vi "TazeASharg - Copy.vi"() -> ()   [LabVIEW 2022 SP3]
uses:
  StopControl.ctl
  StartControl.ctl
  ScoreIndicator.ctl
  TimeControl.ctl
  ComboIndicator.ctl
  NameControl.ctl
  FullHighscoreIndicator.ctl
  HighscoreIndicator.ctl
  FullHighScoreScoreIndicator.ctl
  HighscoreIndicatorYes.ctl
  ShargStates.ctl
  ShargTypeDef.ctl
  <vilib>/numeric/Random Number (Range) U64.vi
  <vilib>/numeric/sub_Random U32.vi
  <vilib>/MakerHub/LINX/Public/Utilities/Open Serial.vi
  <vilib>/MakerHub/LINX/Public/Sensors/Motion/Servo/Servo Open One Channel.vi
  <vilib>/MakerHub/LINX/Public/Sensors/Motion/Servo/Servo Close One Channel.vi
  <vilib>/MakerHub/LINX/LMH-LINX.lvlib
  <vilib>/MakerHub/LINX/Public/Sensors/Motion/Servo/Servo.lvlib
  <vilib>/MakerHub/LINX/Public/Peripherals/PWM/PWM Set Duty Cycle N Chans.vi
panel:
  out "High Score Scores":T1 caption="HIGH SCORE"
  out "High Score Names":T3 caption="HIGH SCORE"
  in  "Name":T5 caption="NAME"
  out "Overheat":bool
  out "COMBO":T6 format="%01d"
  out "TIME":T7 format="%02d"
  out "Hit?":bool
  out "SCORE":T8 format="%04d"
  in  "Start Game":T9
  in  "Stop Button":T10
  out "Energy":dbl(knob) caption="LASER ENERGY" scale=0.0..180.0
  # "HIGH SCORE"
  # "1."
  # "2."
  # "3."
  # "4."
  # "5."
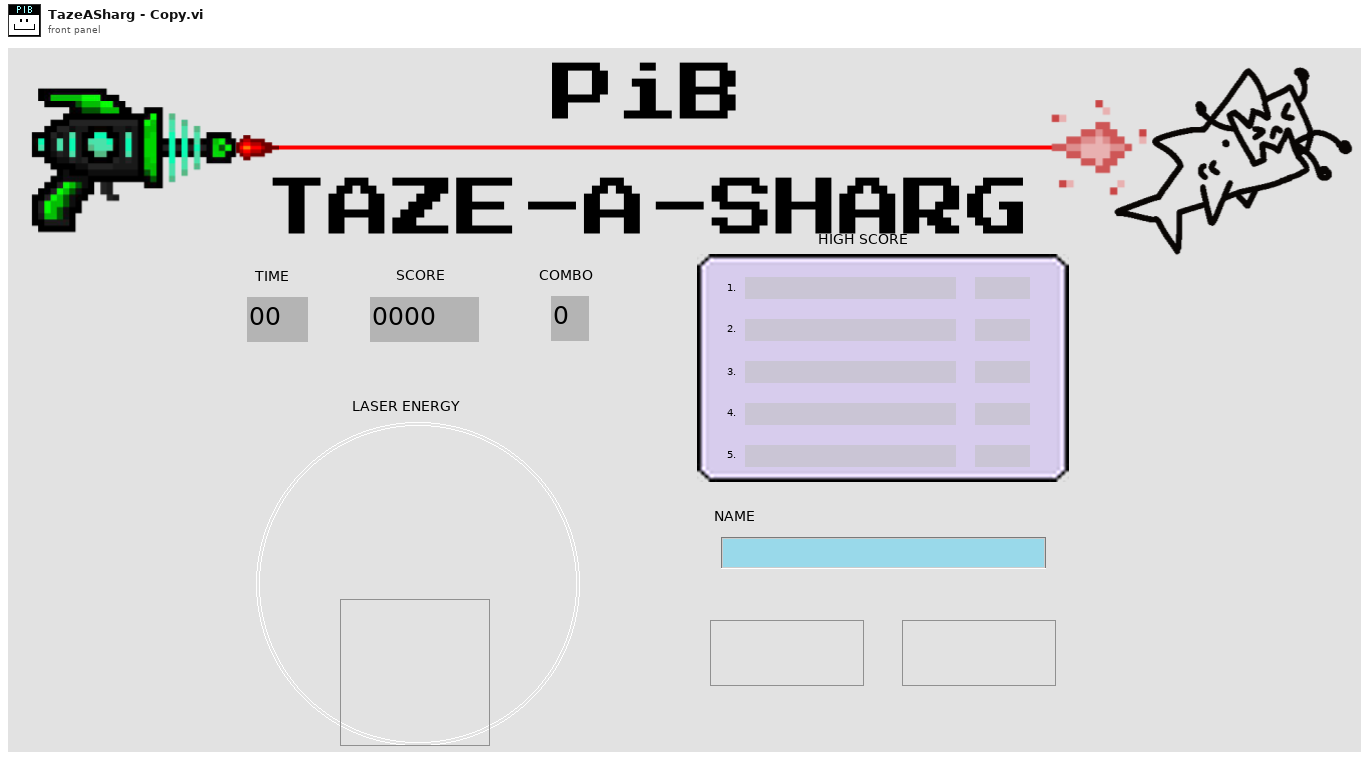
[diagram p1: front panel]
types:
  T1 = typedef "FullHighScoreScoreIndicator.ctl" = T2[]
  T2 = typedef "HighscoreIndicatorYes.ctl" = string
  T3 = typedef "FullHighscoreIndicator.ctl" = T4[]
  T4 = typedef "HighscoreIndicator.ctl" = string
  T5 = typedef "NameControl.ctl" = string
  T6 = typedef "ComboIndicator.ctl" = u32
  T7 = typedef "TimeControl.ctl" = u32
  T8 = typedef "ScoreIndicator.ctl" = u32
  T9 = typedef "StartControl.ctl" = bool
  T10 = typedef "StopControl.ctl" = bool
  T11 = cluster{"Target Up":bool, "Target Start Time":u32, "Target Up Time":u64, "Current Target":u64}
  T12 = cluster{"Laser Pin":u8, "Trigger Pin":u8, "Servo Pin":u8, "Photoresistor Pins":u8[], "RGB LED Pins":u8[]}
  T13 = typedef "ShargStates.ctl" = enum16{"Initialization", "Leaderboard", "Start Game", "Gameplay", "Update Final Score"}
  T14 = typedef "LMH-LINX.lvlib/LINX Ref.ctl" = cluster{"IO":T15, "Interface":T16, "LINX Device Config":T17}
  T15 = typedef "LMH-LINX.lvlib/Platform.ctl" = enum16{"Remote", "Local"}
  T16 = typedef "LMH-LINX.lvlib/Interface.ctl" = enum16{"Serial", "TCP"}
  T17 = typedef "LMH-LINX.lvlib/Device.lvlib/LINX Device Config.ctl" = cluster{"Interface":T16, "COM Port":refnum<visa-resource-name>, "TCP Configuration":T18, "Device Family":u8, "Device ID":u8, "Device Name":string, "TCP Ref":refnum<k5>, "Channels":T19}
  T18 = typedef "LMH-LINX.lvlib/Device.lvlib/TCP Config.ctl" = cluster{"IP Address":string, "Port":u16}
  T19 = typedef "LMH-LINX.lvlib/Channels.ctl" = cluster{"DI":u8[], "DO":u8[], "AI":u8[], "AO":u8[], "PWM":u8[], "QE":u8[], "UART":u8[], "I2C 2":u8[], "SPI":u8[], "CAN":u8[], "Servo":u8[], "AI Ref (V)":dbl, "AI Resolution (Bits)":u8, "AO Ref (V)":dbl, "AO Resolution (Bits)":u8}
  T20 = cluster{"Target Up":bool, "millisecond timer value":u32, "number":u64, "Current Target":u64}
  T21 = enum16{"open", "open or create", "create or replace", "create", "open (read-only)"}
  T22 = typedef "ShargTypeDef.ctl" = cluster{"Start Time":u32, "Score":u32, "Combo":u32, "RisingEdge":u32, "FallingEdge":u32, "Duration":u32, "Signal":i16, "NewTarget?":bool, "Username":string, "LastChannel":i32}
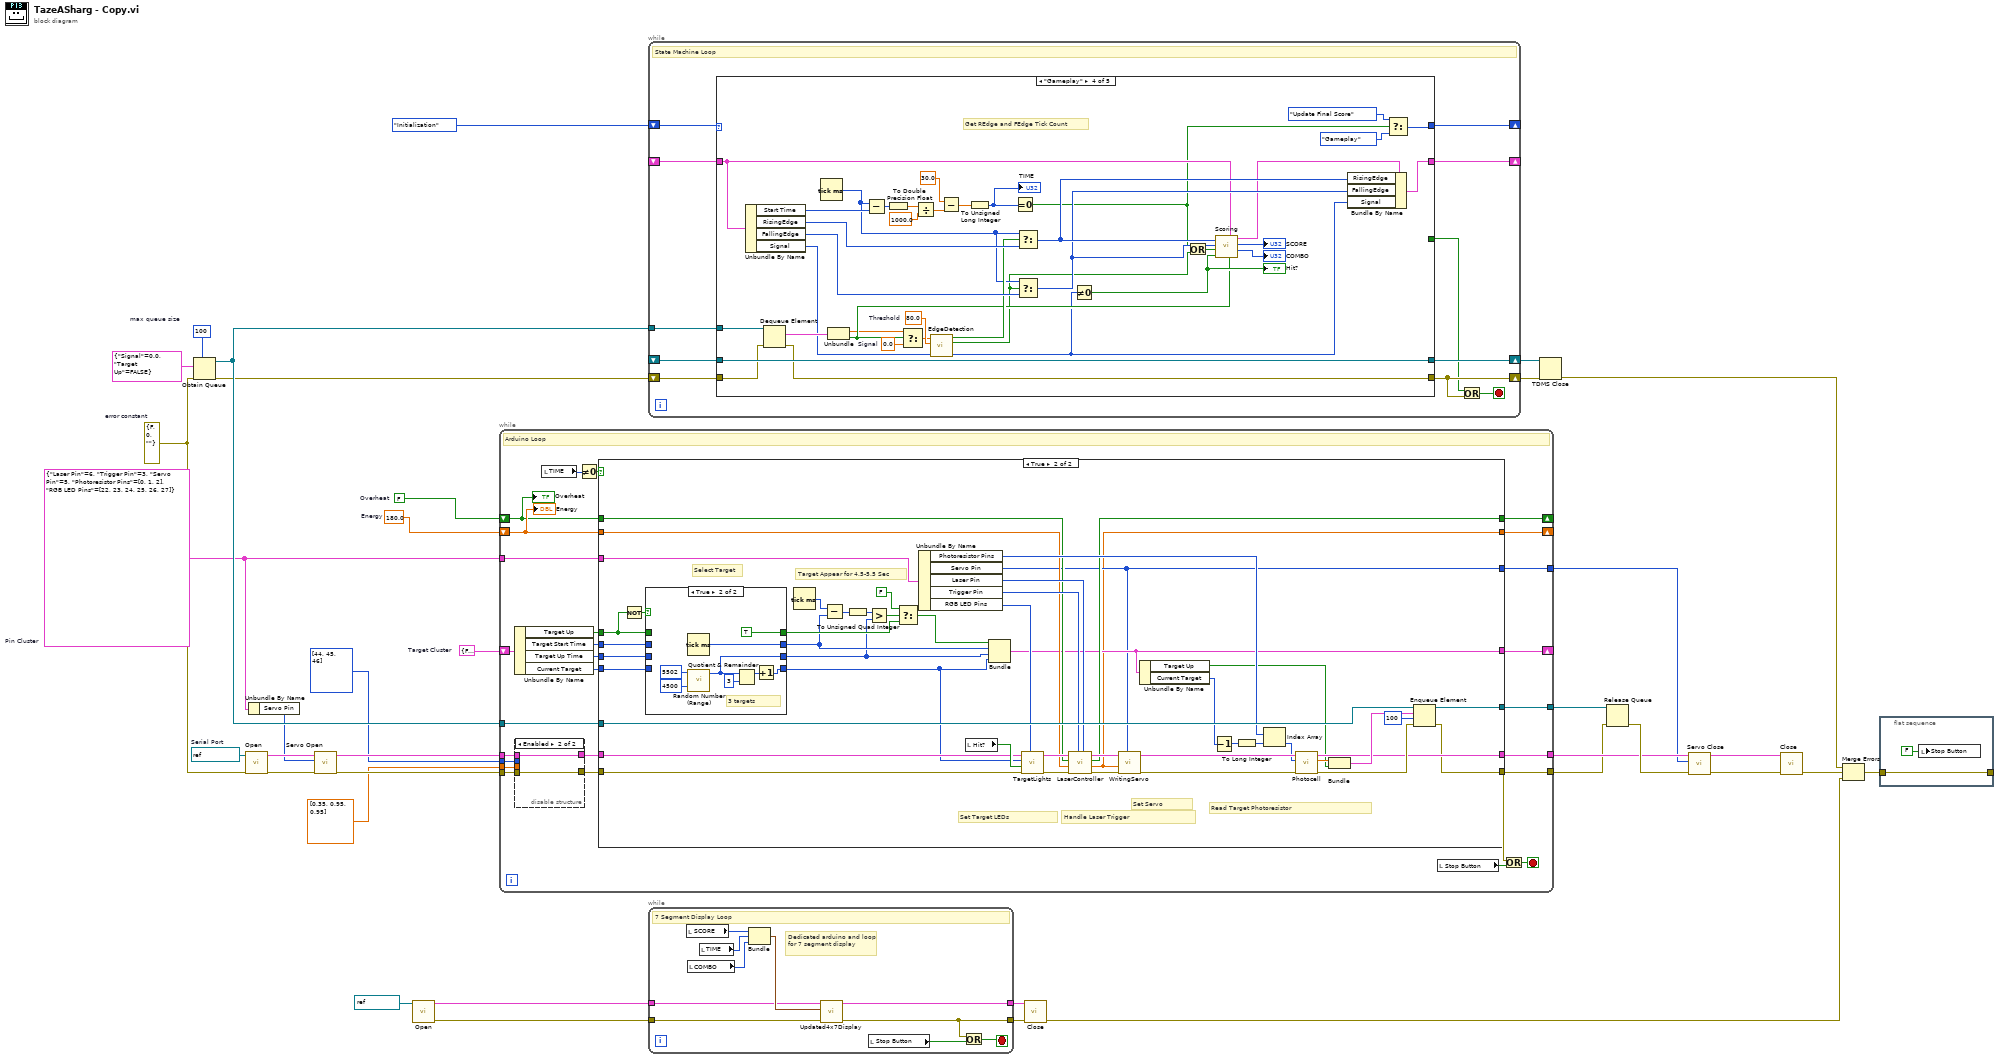
[diagram p0: block diagram]
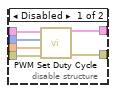
[diagram p2: hidden frame]
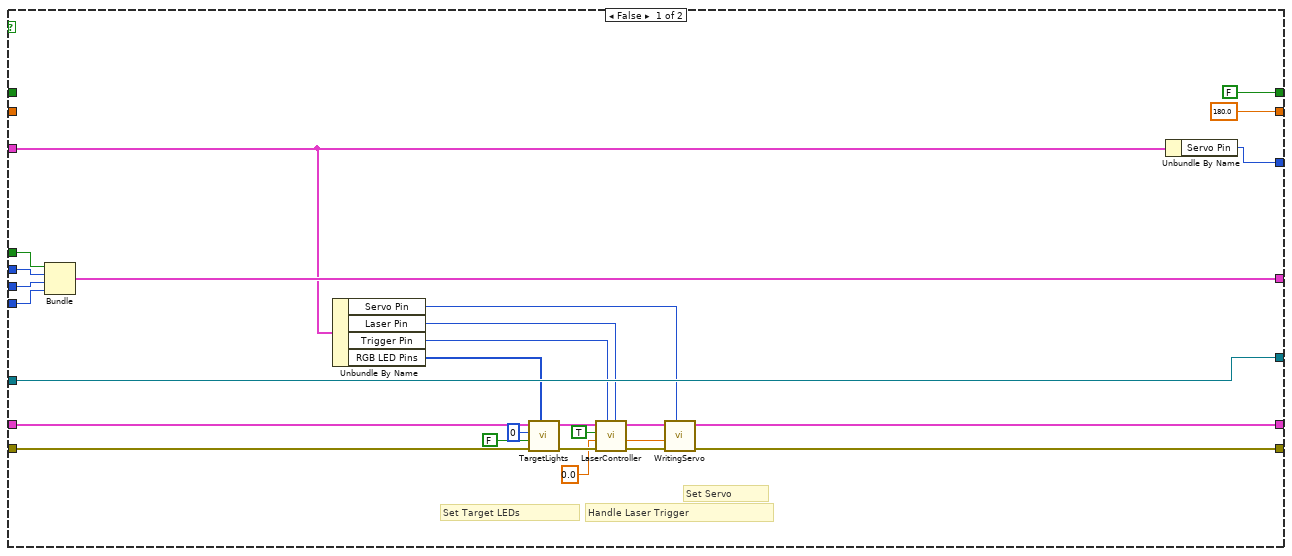
[diagram p3: hidden frame]
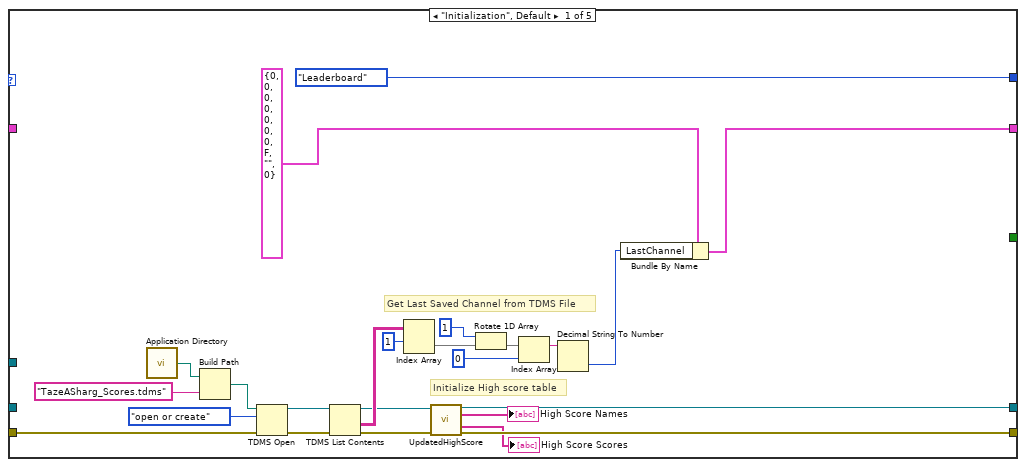
[diagram p5: hidden frame]
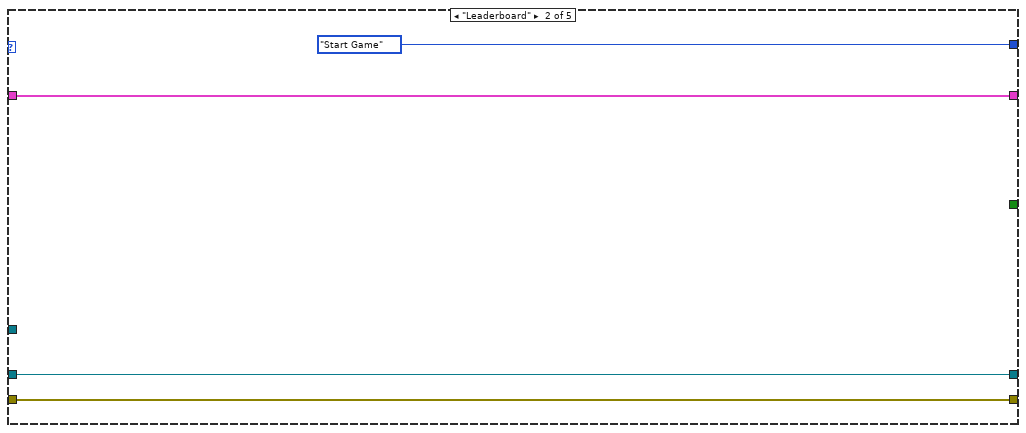
[diagram p6: hidden frame]
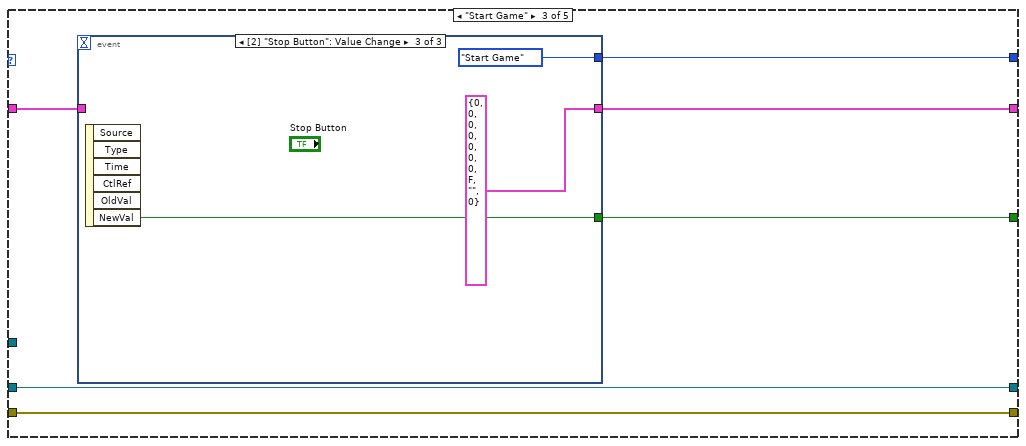
[diagram p7: hidden frame]
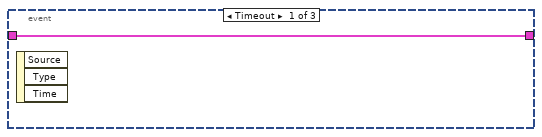
[diagram p8: hidden frame]
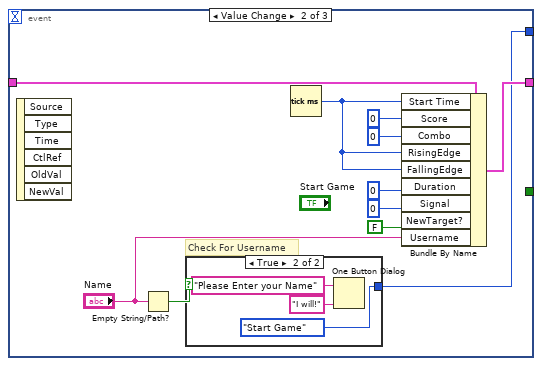
[diagram p9: hidden frame]
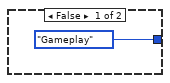
[diagram p10: hidden frame]
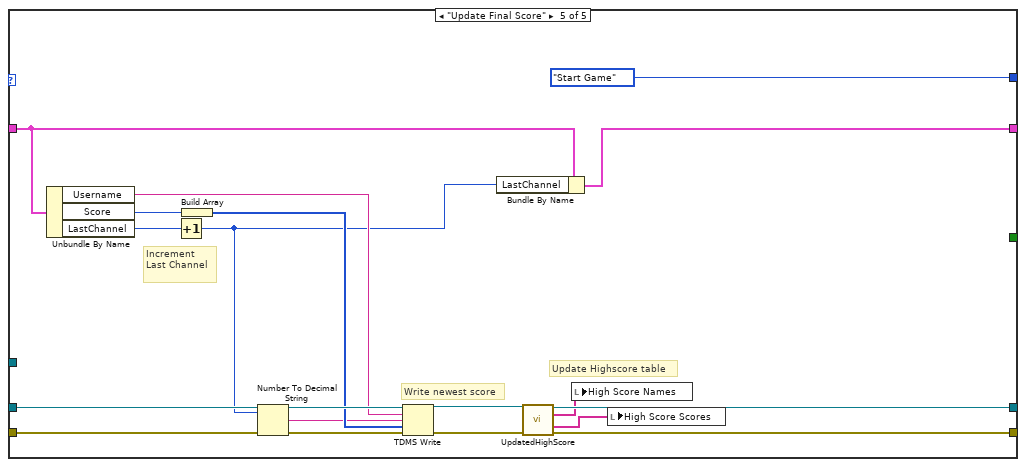
[diagram p11: hidden frame]
diagram:
  w9 = T11 {"Target Up"=FALSE, "Target Start Time"=0, "Target Up Time"=0, "Current Target"=0}  # Target Cluster
  w12 = 180.0  # Energy
  w13 = FALSE  # Overheat
  w6 = T12 {"Laser Pin"=6, "Trigger Pin"=3, "Servo Pin"=5, "Photoresistor Pins"=[0, 1, 2], "RGB LED Pins"=[22, 23, 24, 25, 26, 27]}  # Pin Cluster
  w32 = refnum<visa-resource-name> "COM11"  # Serial Port
  w33 = 100  # max queue size
  w14 = errorcluster {"status"=FALSE, "code"=0, "source"=""}  # error constant
  n1 = Obtain Queue(max queue size (-1, unlimited)=w33, element data type=cluster{"Signal":dbl, "Target Up":bool} {"Signal"=0.0, "Target Up"=FALSE}, error in (no error)=w14) -> (queue out=w35:refnum<queue>, error out=w15:errorcluster)  [unwired: 2 in, 1 out]
  n2 = call-poly <vilib>:"Open.vi"("Error In"=w14, "Serial Port"=w32) -> ("Error Out"=w30:errorcluster, "LINX Resource"=w31:T14)  [unwired: 7 in, 1 out]
  n3 = Unbundle By Name(w6) -> ("Servo Pin"=w5:u8)
  n4 = call-poly <vilib>:"Servo Open.vi"("Error In"=w30, "Servo Channel"=w5, "LINX Resource"=w31) -> ("Error Out"=w4:errorcluster, "LINX Resource"=w3:T14)  [unwired: 7 in]
  n5 = call-poly <vilib>:"Open.vi"("Serial Port"=refnum<visa-resource-name> "COM4") -> ("Error Out"=w24:errorcluster, "LINX Resource"=w25:T14)  [unwired: 8 in, 1 out]
  n6 = while {
    shift-right: [w56] -> _
    shift-left: w13 -> [w53]
    shift-right: [w55] -> _
    shift-left: w12 -> [w54]
    tunnel: w35 -> [w58]
    tunnel: w6 -> [w57]
    tunnel: [w52] -> w11
    tunnel: [w43] -> w7
    tunnel: [w51] -> w10
    shift-right: [w45] -> _
    shift-left: w9 -> [w50]
    tunnel: [w44] -> w8
    tunnel: w4 -> [w40]
    tunnel: w3 -> [w39]
    tunnel: u8[] [44, 45, 46] ("PWM Channels") -> [w38]
    tunnel: dbl[] [0.35, 0.95, 0.95] ("Duty Cycles") -> [w37]
    stop <- w60 stop-if-true
    # "Arduino Loop"
    n7 = Unbundle By Name(w50) -> ("Target Up"=w49:bool, "Target Start Time"=w48:u32, "Target Up Time"=w47:u64, "Current Target"=w46:u64)
    n8 = disable-structure shown="Enabled" {
      disable-tunnel: [w68 w70] -> w42
      disable-tunnel: [w67 w69] -> w41
      disable-tunnel: w40 -> [w66 w69]
      disable-tunnel: w39 -> [w65 w70]
      disable-tunnel: w38 -> [w64 _]
      disable-tunnel: w37 -> [w63 _]
      frame Disabled {
        n9 = call-poly <vilib>:"PWM Set Duty Cycle.vi"("Error In"=w66, "Duty Cycles"=w63, "PWM Channels"=w64, "LINX Resource"=w65) -> ("Error Out"=w67:errorcluster, "LINX Resource"=w68:T14)  [unwired: 6 in]
      }
      frame Enabled {
      }
    }
    n10 = local read "TIME"() -> (w62:T7)
    n11 = Not Equal To 0?(x=w62) -> (x != 0?=w61:bool)
    n12 = case shown="True" w61 {
      tunnel: w48 -> [w93 w140]
      tunnel: w49 -> [w94 w139]
      tunnel: w46 -> [w91 w138]
      tunnel: w47 -> [w92 w137]
      tunnel: w42 -> [w80 w121]
      tunnel: w41 -> [w79 w120]
      tunnel: [w82 w119] -> w52
      tunnel: [w81 w118] -> w43
      tunnel: w58 -> [w95 w117]
      tunnel: w57 -> [w78 w115]
      tunnel: w54 -> [_ w110]
      tunnel: w53 -> [_ w109]
      tunnel: [FALSE ("Overheat Out") w108] -> w56
      tunnel: [180.0 ("Energy Out") w98] -> w55
      tunnel: [w95 w107] -> w51
      tunnel: [w90 w102] -> w45
      tunnel: [w89 w100] -> w44
      frame False {
        # "Set Servo"
        # "Handle Laser Trigger"
        # "Set Target LEDs"
        n13 = Bundle("Target Up"=w94, "Target Start Time"=w93, "Target Up Time"=w92, "Current Target"=w91) -> (w90:T11)  [unwired: 1 in]
        n14 = Unbundle By Name(w78) -> ("Servo Pin"=w74:u8, "Laser Pin"=w75:u8, "Trigger Pin"=w76:u8, "RGB LED Pins"=w77:u8[])
        n15 = call "TargetLights.vi"("DO Channels"=w77, "Error In"=w79, "Hit?"=FALSE, "Target Number"=u64 0, "LINX Resource"=w80) -> ("Error Out"=w85:errorcluster, "LINX Resource 2"=w86:T14)  [unwired: 5 in]
        n16 = call "LaserController.vi"("Laser Pin"=w75, "Trigger Pin"=w76, "Error In"=w85, "Energy In"=0.0, "Overheat In"=TRUE, "LINX Resource In"=w86) -> ("Error Out"=w88:errorcluster, "Energy Out"=w83:dbl, "LINX Resource Out"=w87:T14)  [unwired: 2 in, 1 out]
        n17 = call "WritingServo.vi"("Servo Pin"=w74, "error in (no error)"=w88, "Position"=w83, "LINX Resource in"=w87) -> ("error out"=w81:errorcluster, "LINX Resource out"=w82:T14)  [unwired: 6 in]
        n18 = Unbundle By Name(w78) -> ("Servo Pin"=w89:u8)
      }
      frame True {
        # "Set Servo"
        # "Read Target Photoresistor"
        # "Handle Laser Trigger"
        # "Set Target LEDs"
        # "Target Appear for 4.5-5.5 Sec"
        # "Select Target"
        n19 = Not(x=w139) -> (.not. x?=w136:bool)
        n20 = case shown="True" w136 {
          tunnel: [w148 TRUE] -> w142
          tunnel: [w149 w156] -> w105
          tunnel: [w147 w151] -> w103
          tunnel: w140 -> [w149 _]
          tunnel: w139 -> [w148 _]
          tunnel: w138 -> [w147 _]
          tunnel: [w146 w150] -> w104
          tunnel: w137 -> [w146 _]
          frame False {
          }
          frame True {
            # "3 targets"
            n21 = Tick Count (ms)() -> (millisecond timer value=w156:u32)
            n22 = call-poly <vilib>:"Random Number (Range).vi"("lower bound (0)"=u64 4500, "upper bound (100)"=u64 5502) -> ("number"=w150:u64)  [unwired: 9 in]
            n23 = Quotient & Remainder(x=w150, y=u64 3) -> (x-y*floor(x/y)=w153:u64)  [unwired: 1 out]
            n24 = Increment(x=w153) -> (x+1=w151:u64)
          }
        }
        n25 = Tick Count (ms)() -> (millisecond timer value=w145:u32)
        n26 = Subtract(x=w145, y=w105) -> (x-y=w144:u32)
        n27 = To Unsigned Quad Integer(1:w144) -> (0:w135:u64)
        n28 = Greater?(x=w135, y=w104) -> (0:w143:bool)
        n29 = Select(t=FALSE, s=w143, f=w142) -> (s? t:f=w106:bool)
        n30 = Unbundle By Name(w115) -> ("Photoresistor Pins"=w111:u8[], "Servo Pin"=w100:u8, "Laser Pin"=w112:u8, "Trigger Pin"=w113:u8, "RGB LED Pins"=w114:u8[])
        n31 = local read "Hit?"() -> (w128:bool)
        n32 = Bundle("Target Up"=w106, "millisecond timer value"=w105, "number"=w104, "Current Target"=w103) -> (w102:T20)  [unwired: 1 in]
        n33 = call "TargetLights.vi"("DO Channels"=w114, "Error In"=w120, "Hit?"=w128, "Target Number"=w103, "LINX Resource"=w121) -> ("Error Out"=w125:errorcluster, "LINX Resource 2"=w126:T14)  [unwired: 5 in]
        n34 = call "LaserController.vi"("Laser Pin"=w112, "Trigger Pin"=w113, "Error In"=w125, "Energy In"=w110, "Overheat In"=w109, "LINX Resource In"=w126) -> ("Error Out"=w134:errorcluster, "Energy Out"=w98:dbl, "Overheat Out"=w108:bool, "LINX Resource Out"=w133:T14)  [unwired: 2 in]
        n35 = call "WritingServo.vi"("Servo Pin"=w100, "error in (no error)"=w134, "Position"=w98, "LINX Resource in"=w133) -> ("error out"=w131:errorcluster, "LINX Resource out"=w130:T14)  [unwired: 6 in]
        n36 = Unbundle By Name(w102) -> ("Target Up"=w99:bool, "Current Target"=w101:u64)
        n37 = Decrement(x=w101) -> (x-1=w129:u64)
        n38 = To Long Integer(number=w129) -> (32bit integer=w127:i32)
        n39 = Index Array(array=w111, index=w127) -> (element=w116:u8)
        n40 = call <vilib>:"Photocell.vi"("Error In"=w131, "AI Channel"=w116, "LINX Resource"=w130) -> ("Error Out"=w132:errorcluster, "Value (0-100)"=w123:dbl, "LINX Resource"=w119:T14)  [unwired: 6 in]
        n41 = Bundle("Value (0-100)"=w123, "Target Up"=w99) -> (w124:cluster{"Value (0-100)":dbl, "Target Up":bool})  [unwired: 1 in]
        n42 = Enqueue Element(queue=w117, element=w124, timeout in ms (-1)=100, error in (no error)=w132) -> (queue out=w107:refnum<queue>, error out=w118:errorcluster)  [unwired: 1 out]
      }
    }
    n43 = local read "Stop Button"() -> (w59:T10)
    n44 = Or(x=w43, y=w59) -> (x .or. y?=w60:T10)
    "Overheat" <- w53
    "Energy" <- w54
  }
  n45 = while {
    shift-right: [w167] -> _
    shift-left: ShargStates."Initialization" -> [w168]
    shift-right: [w166] -> _
    shift-left: _ -> [w165]
    tunnel: w35 -> [w164]
    shift-right: [w162] -> w21
    shift-left: _ -> [w161]
    shift-right: [w159] -> w20
    shift-left: w15 -> [w160]
    stop <- w163 stop-if-true
    # "State Machine Loop"
    n46 = case shown="\"Gameplay\"" w168 {
      tunnel: [ShargStates."Leaderboard" ShargStates."Start Game" w202 w259 ShargStates."Start Game"] -> w167
      tunnel: [w171 w195 w200 w222 w260] -> w166
      tunnel: w165 -> [_ w195 w201 w247 w262]
      tunnel: w164 -> [_ _ _ w256 _]
      tunnel: [w174 w193 w199 w223 w266] -> w159
      tunnel: [w175 w194 w197 w228 w267] -> w162
      tunnel: w161 -> [_ w194 w197 w228 w275]
      tunnel: w160 -> [w188 w193 w199 w224 w274]
      tunnel: [_ _ w198 _ _] -> w158
      frame "Initialization", Default {
        # "Get Last Saved Channel from TDMS File"
        # "Initialize High score table"
        n47 = call <vilib>:"Application Directory.vi"() -> ("Application Directory"=w191:path)
        n48 = Build Path(base path=w191, name or relative path="TazeASharg_Scores.tdms") -> (appended path=w190:path)
        n49 = TDMS Open(8:w188, 10:T21."open or create" ("operation (0:open)"), 11:w190) -> (0:w186:errorcluster, 3:w187:refnum<k34>)  [unwired: 4 in]
        n50 = TDMS List Contents(4:w186, 7:w187) -> (0:w173:errorcluster, 1:w180:string[][], 3:w176:refnum<k34>)  [unwired: 1 in, 1 out]
        n51 = Index Array(array=w180, index (row)=1) -> (element=w185:string[])  [unwired: 1 in]
        n52 = call "UpdatedHighScore.vi"("tdms file"=w176, "error in (no error)"=w173) -> ("tdms file out"=w175:refnum<k34>, "Names"=→"High Score Names":string[], "Scores"=→"High Score Scores":string[], "error out"=w174:errorcluster)  [unwired: 10 in]
        n53 = Rotate 1D Array(1:w185, 2:1 ("n")) -> (0:w183:string[])
        n54 = Index Array(array=w183, index=0) -> (element=w179:string)
        n55 = Decimal String To Number(string=w179) -> (number=w177:i32)  [unwired: 2 in, 1 out]
        n56 = Bundle By Name(cluster=T22 {"Start Time"=0, "Score"=0, "Combo"=0, "RisingEdge"=0, "FallingEdge"=0, "Duration"=0, "Signal"=0, "NewTarget?"=FALSE, "Username"="", "LastChannel"=0} ("Cluster"), "LastChannel"=w177) -> (w171:T22)
      }
      frame "Leaderboard" {
      }
      frame "Start Game" {
        n57 = event shown="[2] \"Stop Button\": Value Change" {
          selector: _ -> [_ _ _]
          dyn-events: _ -> [_ _ _]
          timeout: _ -> [_ _ _]
          tunnel: [_ w205 ShargStates."Start Game"] -> w202
          tunnel: w201 -> [w203 w214 _]
          tunnel: [w203 w213 T22 {"Start Time"=0, "Score"=0, "Combo"=0, "RisingEdge"=0, "FallingEdge"=0, "Duration"=0, "Signal"=0, "NewTarget?"=FALSE, "Username"="", "LastChannel"=0} ("Cluster Out")] -> w200
          tunnel: [_ _ w219] -> w198
          event Timeout {
            n58 = event-data() -> ()  [unwired: 1 in, 3 out]
          }
          event Value Change {
            # "Check For Username"
            n59 = event-data() -> ()  [unwired: 1 in, 6 out]
            n60 = Empty String/Path?(string/path="Name") -> (empty?=w206:bool)
            n61 = case shown="True" w206 {
              tunnel: [ShargStates."Gameplay" ShargStates."Start Game"] -> w205
              frame False {
              }
              frame True {
                n62 = One Button Dialog(message="Please Enter your Name", button name ("OK")="I will!") -> ()  [unwired: 1 out]
              }
            }
            n63 = Tick Count (ms)() -> (millisecond timer value=w207:u32)
            n64 = Bundle By Name(cluster=w214, "Start Time"=w207, "Score"=u32 0, "Combo"=u32 0, "RisingEdge"=w207, "FallingEdge"=w207, "Duration"=u32 0, "Signal"=i16 0, "NewTarget?"=FALSE, "Username"="Name") -> (w213:T22)
          }
          event Value Change {
            n65 = event-data() -> ("NewVal"=w219:T10)  [unwired: 1 in, 5 out]
          }
        }
      }
      frame "Gameplay" {
        w249 = 0.0  # Signal
        w255 = 80.0  # Threshold
        # "Get REdge and FEdge Tick Count"
        n66 = Unbundle By Name(w247) -> ("Start Time"=w245:u32, "RisingEdge"=w252:u32, "FallingEdge"=w251:u32, "Signal"=w231:i16)
        n67 = Dequeue Element(queue=w256, error in (no error)=w224) -> (element=w246:cluster{"Signal":dbl, "Target Up":bool}, error out=w223:errorcluster)  [unwired: 1 in, 2 out]
        n68 = Tick Count (ms)() -> (millisecond timer value=w244:u32)
        n69 = Unbundle(w246) -> ("Signal"=w233:dbl, "Target Up"=w234:bool)
        n70 = Subtract(x=w244, y=w245) -> (x-y=w243:u32)
        n71 = To Double Precision Float(number=w243) -> (double precision float=w241:dbl)
        n72 = Select(t=w233, s=w234, f=w249) -> (s? t:f=w232:dbl)
        n73 = Divide(x=w241, y=1000.0) -> (x/y=w240:dbl)
        n74 = call "EdgeDetection.vi"("Previous Value"=w231, "Threshold"=w255, "Analog Input"=w232) -> ("Digitized"=w230:i16, "Falling Edge"=w226:bool, "Rising Edge"=w250:bool)  [unwired: 4 in]
        n75 = Subtract(x=30.0, y=w240) -> (x-y=w236:dbl)
        n76 = To Unsigned Long Integer(number=w236) -> (unsigned 32bit integer=w229:u32)
        "TIME" <- w229
        n77 = Equal To 0?(x=w229) -> (x = 0?=w227:bool)
        n78 = Select(t=w244, s=w250, f=w252) -> (s? t:f=w254:u32)
        n79 = Select(t=w244, s=w226, f=w251) -> (s? t:f=w253:u32)
        n80 = Not Equal To 0?(x=w230) -> (x != 0?=w235:bool)
        "Hit?" <- w235
        n81 = Or(x=w227, y=w226) -> (x .or. y?=w225:bool)
        n82 = call "Scoring.vi"("RisingEdge"=w254, "FallingEdge"=w253, "FallingEdge?"=w225, "Hit?"=w235, "Cluster In"=w247, "TargetUp?"=w234) -> ("Cluster Out"=w248:T22, "Live Score"=→"SCORE":u32, "Combo"=→"COMBO":u32)  [unwired: 2 in]
        n83 = Bundle By Name(cluster=w248, "RisingEdge"=w254, "FallingEdge"=w253, "Signal"=w230) -> (w222:T22)
        n84 = Select(t=ShargStates."Update Final Score", s=w227, f=ShargStates."Gameplay") -> (s? t:f=w259:T13)
      }
      frame "Update Final Score" {
        # "Write newest score"
        # "Update Highscore table"
        # "Increment Last Channel"
        n85 = Unbundle By Name(w262) -> ("Username"=w270:string, "Score"=w273:u32, "LastChannel"=w269:i32)
        n86 = Increment(x=w269) -> (x+1=w261:i32)
        n87 = Build Array(w273) -> (w272:u32[])
        n88 = Number To Decimal String(number=w261) -> (decimal integer string=w271:string)  [unwired: 1 in]
        n89 = TDMS Write(0:w275, 5:w270, 7:w271, 9:w272, 11:w274) -> (4:w268:refnum<k34>, 15:w265:errorcluster)  [unwired: 1 in, 2 out]
        n90 = Bundle By Name(cluster=w262, "LastChannel"=w261) -> (w260:T22)
        n91 = call "UpdatedHighScore.vi"("tdms file"=w268, "error in (no error)"=w265) -> ("tdms file out"=w267:refnum<k34>, "Names"=w264:string[], "Scores"=w263:string[], "error out"=w266:errorcluster)  [unwired: 10 in]
        n92 = local write "High Score Names"(w264) -> ()
        n93 = local write "High Score Scores"(w263) -> ()
      }
    }
    n94 = Or(x=w158, y=w159) -> (x .or. y?=w163:T10)
  }
  n95 = while {
    tunnel: w25 -> [w282]
    tunnel: w24 -> [w281]
    tunnel: [w280] -> w23
    tunnel: [w278] -> w22
    stop <- w279 stop-if-true
    # "Dedicated arduino and loop for 7 segment display"
    # "7 Segment Display Loop"
    n96 = local read "SCORE"() -> (w286:T8)
    n97 = local read "COMBO"() -> (w284:T6)
    n98 = local read "TIME"() -> (w285:T7)
    n99 = Bundle("SCORE"=w286, "TIME"=w285, "COMBO"=w284) -> (w283:cluster{"SCORE":T8, "TIME":T7, "COMBO":T6})  [unwired: 1 in]
    n100 = call "Updated4x7Display.vi"("Error In"=w281, "Cluster"=w283, "LINX Resource In"=w282) -> ("Error Out"=w278:errorcluster, "LINX Resource Out"=w280:T14)  [unwired: 7 in]
    n101 = local read "Stop Button"() -> (w277:T10)
    n102 = Or(x=w278, y=w277) -> (x .or. y?=w279:T10)
  }
  n103 = call <vilib>:"Close.vi"("Error In"=w22, "LINX Resource"=w23) -> ("Error Out"=w16:errorcluster)  [unwired: 9 in]
  n104 = TDMS Close(8:w20, 11:w21) -> (0:w17:errorcluster)  [unwired: 1 out]
  n105 = Release Queue(queue=w10, error in (no error)=w7) -> (error out=w27:errorcluster)  [unwired: 1 in, 2 out]
  n106 = call-poly <vilib>:"Servo Close.vi"("Error In"=w27, "Servo Channel"=w8, "LINX Resource"=w11) -> ("Error Out"=w28:errorcluster, "LINX Resource"=w29:T14)  [unwired: 7 in]
  n107 = call <vilib>:"Close.vi"("Error In"=w28, "LINX Resource"=w29) -> ("Error Out"=w19:errorcluster)  [unwired: 9 in]
  n108 = Merge Errors(w17, w19, w16) -> (w18:errorcluster)
  n109 = flat-sequence {
    tunnel: w18 -> [w287]
    tunnel: [w287] -> _
    frame #0 {
      n110 = local write "Stop Button"(FALSE ("Stop Button")) -> ()
    }
  }
